vi "Basic Level Trigger Detection.vi"   [LabVIEW 2020, in "NI_MAPro.lvlib"]
doc: "Finds the first level-crossing location in a waveform. You can retrieve the trigger location as an index or as a time. The trigger conditions are specified in terms of threshold <B>level</B>, <B>slope</B>, and <B>hysteresis</B>. Wire data to the <B>signal in</B> input to determine the polymorphic instance to use or manually select the instance."
uses:
  NI_MAPro.lvlib
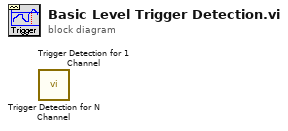
[diagram p0: block diagram]
diagram:
  n1 = call "Trigger Detection for N Channel.vi"() -> ()  [unwired: 13 in, 3 out]
  n2 = call "Trigger Detection for 1 Channel.vi"() -> ()  [unwired: 13 in, 3 out]
